vi "Main - Encrypt (SubVI).vi"(11 "String":string) -> (3 "Base64 String":string)   [LabVIEW 2019]
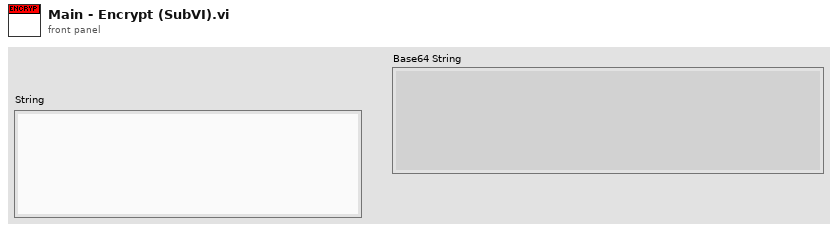
[diagram p1: front panel]
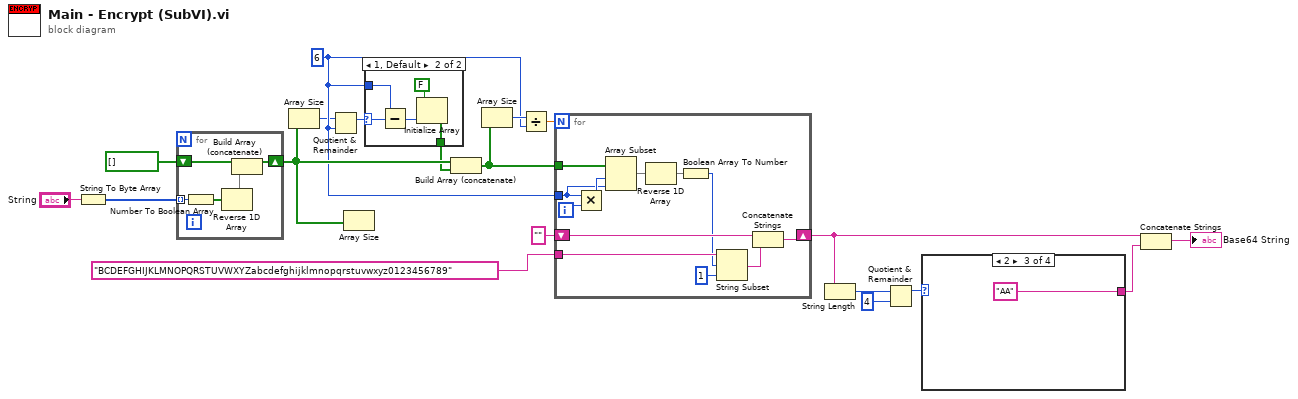
[diagram p0: block diagram]
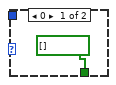
[diagram p2: hidden frame]
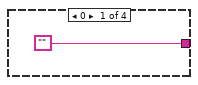
[diagram p3: hidden frame]
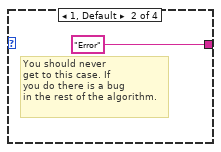
[diagram p4: hidden frame]
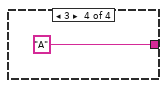
[diagram p5: hidden frame]
diagram:
  w16 = 6 ("y")
  n1 = String To Byte Array(string="String") -> (unsigned byte array=w1:u8[])
  n2 = for {
    tunnel: w1 -> [w24] mode=indexing
    shift-right: [w21] -> w19
    shift-left: bool[] [] -> [w23]
    n3 = Number To Boolean Array(number=w24) -> (Boolean array=w22:bool[])
    n4 = Reverse 1D Array(array=w22) -> (reversed array=w20:bool[])
    n5 = Build Array (concatenate)(w23, w20) -> (w21:bool[])
  }
  n6 = Array Size(array=w19) -> (size(s)=w13:i32)
  n7 = Quotient & Remainder(x=w13, y=w16) -> (x-y*floor(x/y)=w14:i32)  [unwired: 1 out]
  n8 = Array Size(array=w19) -> ()  [unwired: 1 out]
  n9 = case shown="1, Default" w14 {
    selector: w14 -> [_ w29]
    tunnel: [bool[] [] w26] -> w15
    tunnel: w16 -> [_ w28]
    frame 0 {
    }
    frame 1, Default {
      n10 = Subtract(x=w28, y=w29) -> (x-y=w30:i32)
      n11 = Initialize Array(FALSE, w30) -> (w26:bool[])
    }
  }
  n12 = Build Array (concatenate)(w19, w15) -> (w17:bool[])
  n13 = Array Size(array=w17) -> (size(s)=w18:i32)
  n14 = Divide(x=w18, y=w16) -> (x/y=w12:dbl)
  n15 = for {
    N: w12 -> [_]
    tunnel: w17 -> [w41]
    tunnel: w16 -> [w39]
    tunnel: "BCDEFGHIJKLMNOPQRSTUVWXYZabcdefghijklmnopqrstuvwxyz0123456789" -> [w38]
    shift-right: [w36] -> w10
    shift-left: "" -> [w35]
    i -> [w42]
    n16 = Multiply(x=w39, y=w42) -> (x*y=w40:i32)
    n17 = Array Subset(array=w41, index=w40, length=w39) -> (w31:bool[])
    n18 = Reverse 1D Array(array=w31) -> (reversed array=w32:bool[])
    n19 = Boolean Array To Number(Boolean array=w32) -> (number=w33:u32)
    n20 = String Subset(string=w38, offset (0)=w33, length (rest)=1 ("length (rest)")) -> (substring=w34:string)
    n21 = Concatenate Strings(w35, w34) -> (w36:string)
  }
  n22 = String Length(string=w10) -> (length=w6:i32)
  n23 = Quotient & Remainder(x=w6, y=4) -> (x-y*floor(x/y)=w8:i32)  [unwired: 1 out]
  n24 = case shown="2" w8 {
    tunnel: ["" "Error" "AA" "A"] -> w9
    frame 0 {
    }
    frame 1, Default {
      # "You should never\nget to this case. If\nyou do there is a bug\nin the rest of the algorithm."
    }
    frame 2 {
    }
    frame 3 {
    }
  }
  n25 = Concatenate Strings(w10, w9) -> (→"Base64 String":string)
